vi "Phasor Covariance (g, s) for discrete Lambda_tau,T,W(t).vi"(6 "Phasor Frequency":dbl[unit], 8 "Error In":errorcluster, 9 "Photons (100)":i32=100, 10 "Square-Gated Periodic Exponential Parameters":cluster{"t":dbl, "W":dbl, "Period":dbl, "G":i32}={"t"=0.0, "W"=0.0, "Period"=12.5, "G"=100} {"Period" format="%#_13g"}, 11 "# Simulations (100)":i32=100) -> (0 "Error Out":errorcluster, 3 "Covariance":dbl)   [LabVIEW 2021, in "Phasor.lvlib"]
doc: "Computes the covariance of s and g, the phasor components, for a discrete square-gated periodic exponential assuming Poisson-distributed gate intensities.\n\n<B># Simulations</B>: number of simulated decays\n\n<B>Square-Gated Periodic Exponential Parameters</B>: decay parameters. Temporal parameters are assumed to be in ns.\n\n<B>Photons</B>: total average photons in the decay\n\n<B>Phasor Frequency</B>: phasor harmonic frequency"
uses:
  Arrays/Linear Ramp End Options.ctl
  129a87f0-f368-433e-8409-a21c4dac2cf5.vi
  Math/Lambda_tau,T,W 1(s').vi
  Math/Lambda_tau,T,W 2(s').vi
  <vilib>/gmath/statdist.llb/Poisson Random.vi
  Phasor.lvlib
  Arrays/Arrays.lvlib
  <vilib>/gmath/NI_Gmath.lvlib
  <vilib>/Analysis/NI_AALBase.lvlib
  Time/Time.lvlib
  Error/Error.lvlib
panel:
  out "CPU (s)":dbl
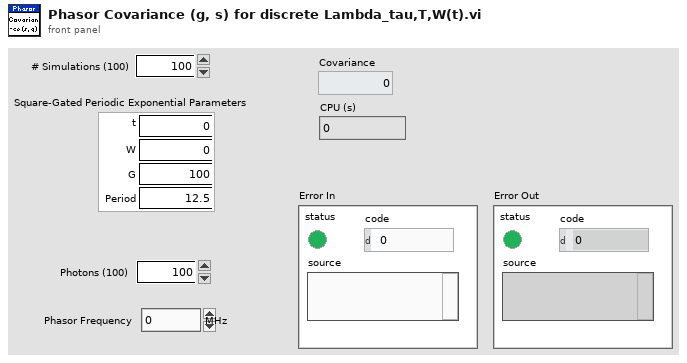
[diagram p1: front panel]
types:
  T1 = typedef "Arrays.lvlib/Linear Ramp End Options.ctl" = enum16{"Include Min/Exclude Max", "Exclude Min/Include Max", "Include Both Ends", "Exclude Both Ends"}
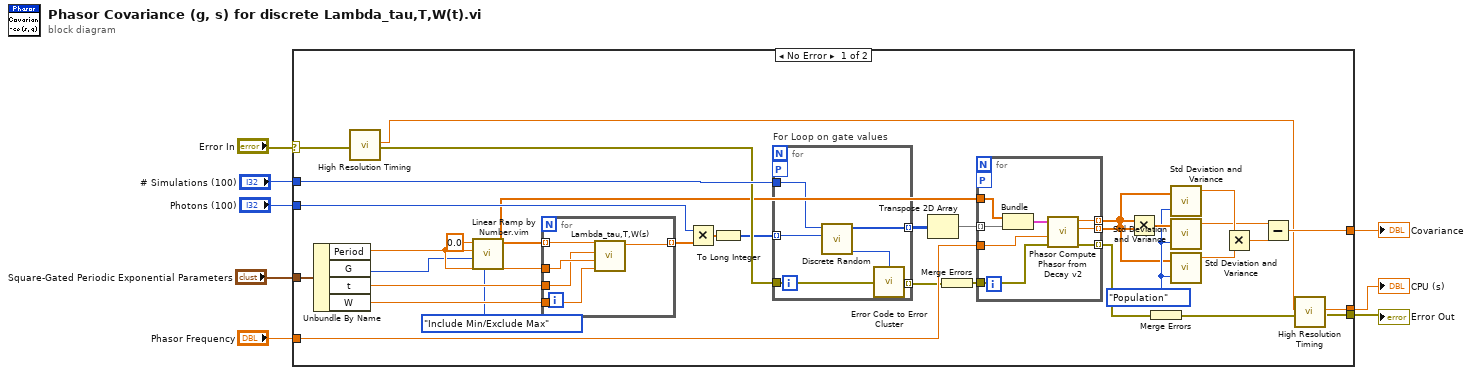
[diagram p0: block diagram]
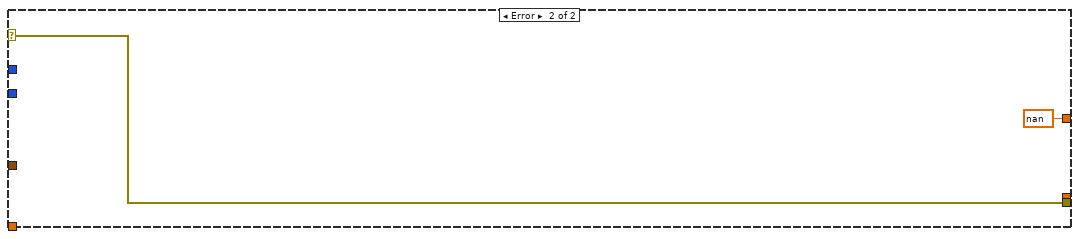
[diagram p2: hidden frame]
diagram:
  n1 = case shown="No Error" "Error In" {
    selector: "Error In" -> [w30 w63]
    tunnel: "Photons (100)" -> [w42 _]
    tunnel: "# Simulations (100)" -> [w41 _]
    tunnel: "Phasor Frequency" -> [w40 _]
    tunnel: [w39 nan] -> w5
    tunnel: [w36 _] -> w4
    tunnel: "Square-Gated Periodic Exponential Parameters" -> [w33 _]
    tunnel: [w28 w63] -> w1
    frame No Error {
      w17 = enum16{"Sample", "Population"}."Population" ("Weighting (Sample)")
      n2 = Unbundle By Name(w33) -> ("Period"=w35:dbl, "G"=w34:i32, "t"=w32:dbl, "W"=w31:dbl)
      n3 = call "High Resolution Timing.vi"("Error In"=w30) -> ("elapsed (relative) seconds"=w37:dbl, "Error Out"=w38:errorcluster)  [unwired: 16 in, 1 out]
      n4 = call "Linear Ramp by Number.vim"("Options"=Linear_Ramp_End_Options."Include Min/Exclude Max", "# Steps (1)"=w34, "End (1)"=w35, "Start (0)"=0.0) -> ("Ramp"=w20:dbl[])  [unwired: 5 in, 2 out]
      n5 = for {
        tunnel: w20 -> [w55] mode=indexing
        tunnel: w35 -> [w54]
        tunnel: [w53] -> w25 mode=indexing
        tunnel: w32 -> [w52]
        tunnel: w31 -> [w51]
        n6 = call "Lambda_tau,T,W(s).vi"("W"=w51, "T"=w54, "t"=w52, "s"=w55) -> ("L_tau,T,W(s)"=w53:dbl)  [unwired: 7 in]
      }
      n7 = Multiply(x=w42, y=w25) -> (x*y=w24:dbl[])
      n8 = To Long Integer(number=w24) -> (32bit integer=w23:i32[])
      n9 = for "For Loop on gate values" {
        tunnel: w23 -> [w60] mode=indexing
        tunnel: w41 -> [w61]
        tunnel: [w59] -> w22 mode=indexing
        workers-P: _ -> [_]
        tunnel: [w57] -> w11 mode=indexing
        tunnel: w38 -> [w56]
        n10 = call-poly <vilib>:"Discrete Random.vi"("lambda"=w60, "samples"=w61) -> ("error"=w58:i32, "Poisson random data"=w59:i32[])  [unwired: 8 in]
        n11 = call "Error Code to Error Cluster.vi"("Error Code"=w58, "Error In"=w56) -> ("Error Out"=w57:errorcluster)  [unwired: 13 in]
      }
      n12 = Transpose 2D Array(2D array=w22) -> (transposed array=w21:i32[][])
      n13 = Merge Errors(w11) -> (w10:errorcluster)
      n14 = for {
        tunnel: w21 -> [w49] mode=indexing
        tunnel: w40 -> [w50]
        tunnel: w20 -> [w48]
        tunnel: [w46] -> w18 mode=indexing
        tunnel: [w45] -> w16 mode=indexing
        workers-P: _ -> [_]
        tunnel: w10 -> [w44]
        tunnel: [w43] -> w9 mode=indexing
        n15 = Bundle("Ramp"=w48, w49) -> (w47:cluster{"Ramp":dbl[], i32[]})  [unwired: 1 in]
        n16 = call "Phasor Compute Phasor from Decay v2.vi"("Error In"=w44, "Phasor Frequency"=w50, "Time-Gated Decay"=w47) -> ("Error Out"=w43:errorcluster, "s"=w45:dbl, "g"=w46:dbl)  [unwired: 5 in, 1 out]
      }
      n17 = Multiply(x=w18, y=w16) -> (x*y=w19:dbl[])
      n18 = Merge Errors(w9) -> (w29:errorcluster)
      n19 = call <vilib>:"Std Deviation and Variance.vi"("X"=w18, "Weighting (Sample)"=w17) -> ("mean"=w14:dbl)  [unwired: 2 out]
      n20 = call <vilib>:"Std Deviation and Variance.vi"("X"=w19, "Weighting (Sample)"=w17) -> ("mean"=w13:dbl)  [unwired: 2 out]
      n21 = call <vilib>:"Std Deviation and Variance.vi"("X"=w16, "Weighting (Sample)"=w17) -> ("mean"=w15:dbl)  [unwired: 2 out]
      n22 = Multiply(x=w14, y=w15) -> (x*y=w12:dbl)
      n23 = Subtract(x=w13, y=w12) -> (x-y=w39:dbl)
      n24 = call "High Resolution Timing.vi"("relative seconds (NaN)"=w37, "Error In"=w29) -> ("elapsed (relative) seconds"=w36:dbl, "Error Out"=w28:errorcluster)  [unwired: 15 in, 1 out]
    }
    frame Error {
    }
  }
  "Covariance" <- w5
  "CPU (s)" <- w4
  "Error Out" <- w1
